vi "TCL Global.vi"() -> ()   [LabVIEW 2009]
panel:
  in  "Fragments":string[](array[string])
  in  "Current BaseFile Name":path
  in  "Current EventFile Name":path
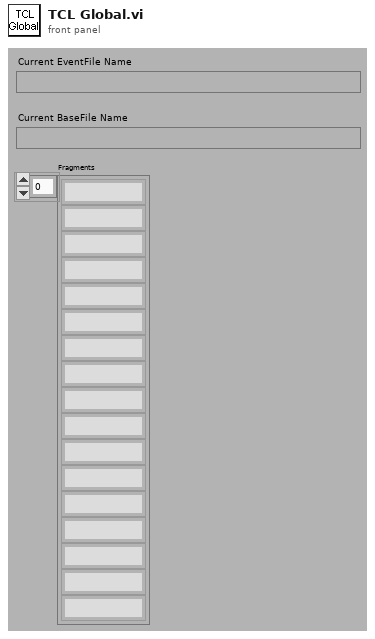
[diagram p1: front panel]
diagram:
